vi "AO_single_FPGA.vi"() -> ()   [LabVIEW 2021]
uses:
  <vilib>/rvi/Emulation/niFpgaGetClockAttributes.vi
  <vilib>/rvi/Emulation/niFpgaSctlEmulationGetInTimedLoop.vi
  <vilib>/rvi/Emulation/niFpgaEmulationReportErrorSimple.vi
  <vilib>/rvi/Emulation/niFpgaProcessEmulError.vi
  <vilib>/rvi/interface/RandomDataEmulation/niFpgaRandomDataHandleErrors.vi
  <vilib>/rvi/Emulation/niFpgaCriticalErrorInLSC.vi
  <vilib>/rvi/eio/common/nirviEmuTemplateMethod_errors.vi
  <vilib>/rvi/DataTransferAndStorage/Container/XNode/niFpgaContainer.xnode
  <vilib>/rvi/interface/RandomDataEmulation/nirviRandomDataFpgaReadWriteTemplate.vi
  <vilib>/eio/EIONode/EIONode.xnode
panel:
  in  "AO Enable":bool
  in  "AO 0":sgl
  in  "AO 1":sgl
  in  "AO 2":sgl
  in  "AO 3":sgl
  in  "AO 4":sgl
  in  "AO 5":sgl
  in  "AO 6":sgl
  in  "AO 7":sgl
  in  "AO Loop Timer (ticks)":i32
  out "AO: Actual Loop Rate (ticks)":u32
  out "AO Buffer Underflow?":bool
  in  "AO Buffer Enable":u8 format="%08b"
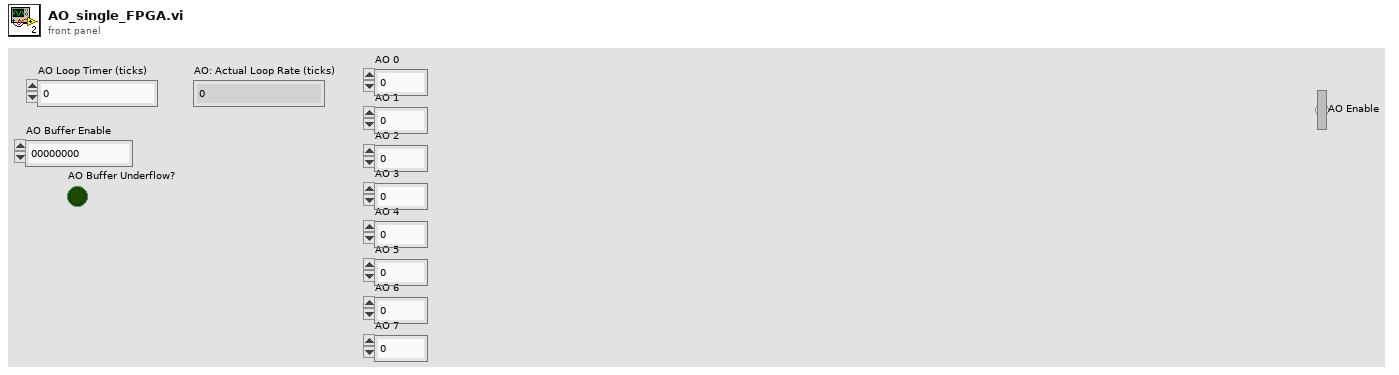
[diagram p1: front panel]
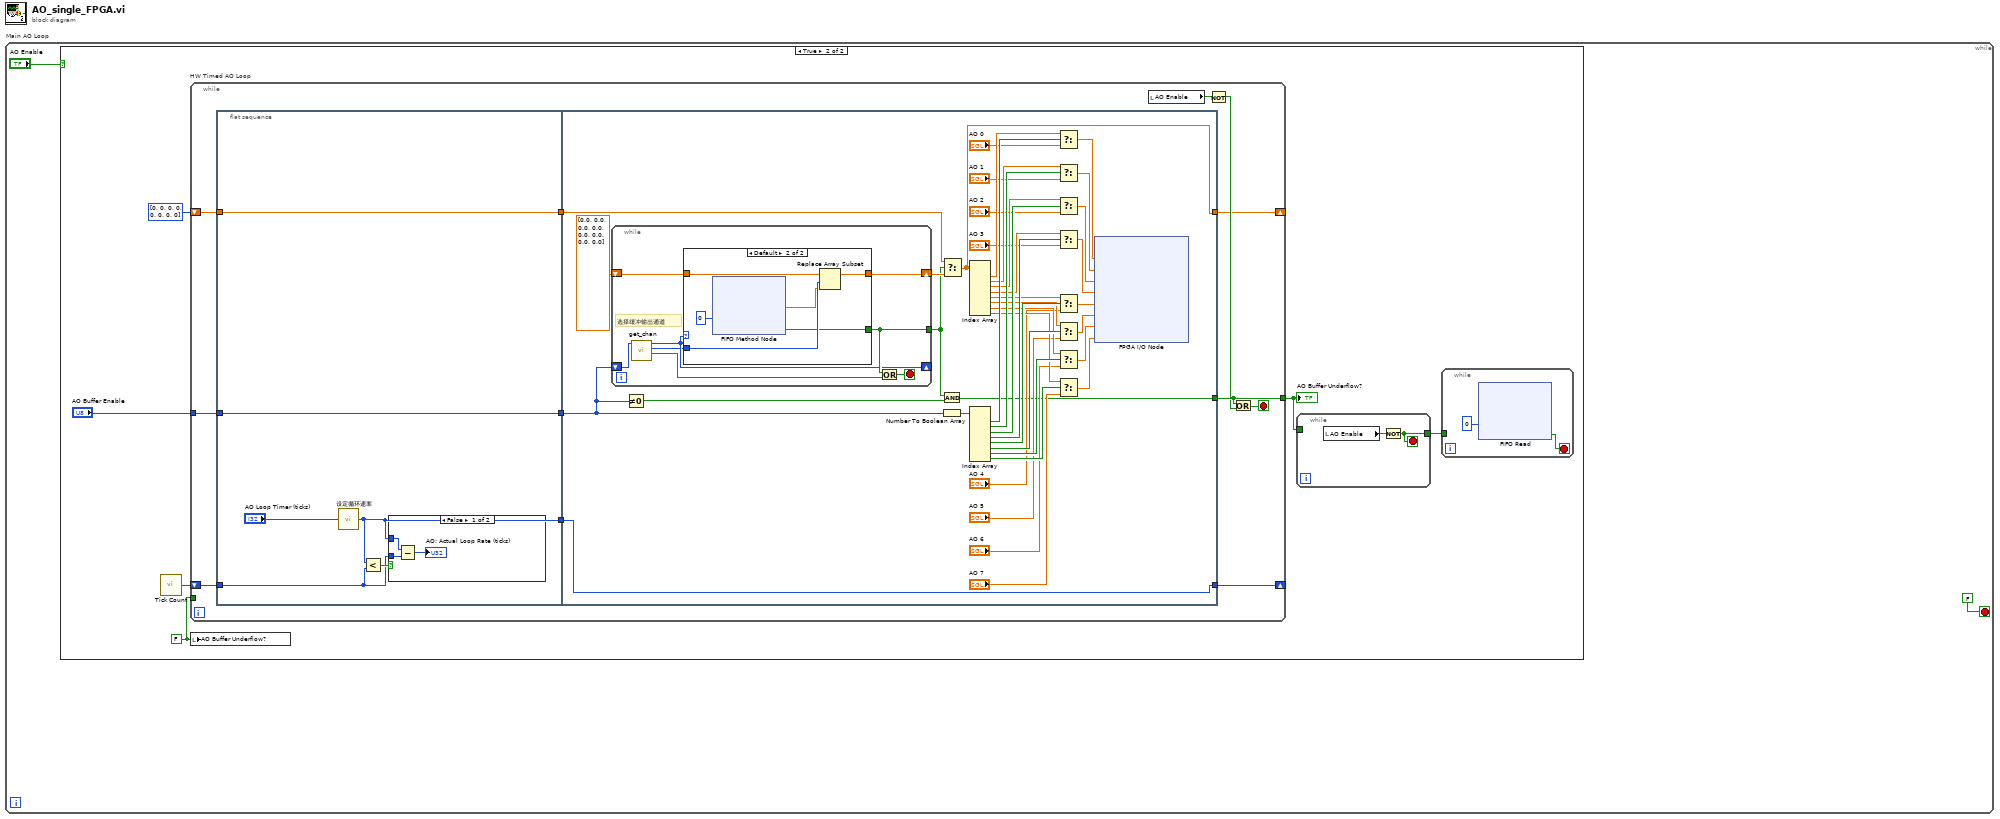
[diagram p0: block diagram]
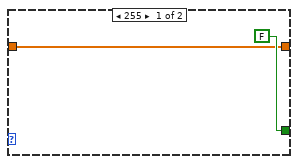
[diagram p4: hidden frame]
diagram:
  n1 = while "Main AO Loop" {
    stop <- FALSE stop-if-true
    n2 = case shown="True" "AO Enable" {
      frame False {
      }
      frame True {
        w8 = FALSE ("AO Buffer Underflow?")
        n3 = call "Tick Count"() -> ("Tick Count(Ticks)"=w3:u32)
        n4 = while "HW Timed AO Loop" {
          tunnel: [w23] -> w5
          tunnel: w8 -> [_]
          tunnel: "AO Buffer Enable" -> [w20]
          shift-right: [w18] -> _
          shift-left: i16[] [0, 0, 0, 0, 0, 0, 0, 0] -> [w17]
          shift-right: [w14] -> _
          shift-left: w3 -> [w13]
          stop <- w24 stop-if-true
          n5 = flat-sequence {
            tunnel: w20 -> [w30]
            tunnel: [w30] -> w19
            tunnel: w17 -> [w29]
            tunnel: [w29] -> w16
            tunnel: [w25] -> w15
            tunnel: w13 -> [w27]
            tunnel: [w34] -> w23
            tunnel: w19 -> [w37]
            tunnel: [w71] -> w18
            tunnel: w16 -> [w70]
            tunnel: w15 -> [w38]
            tunnel: [w38] -> w14
            frame #0 {
              n6 = call "设定循环速率"("Count(Ticks)"="AO Loop Timer (ticks)") -> ("Tick Count(Ticks)"=w25:u32)
              n7 = Less?(x=w25, y=w27) -> (x < y?=w28:bool)
              n8 = case shown="False" w28 {
                tunnel: w25 -> [w33 _]
                tunnel: w27 -> [w32 _]
                frame False {
                  n9 = Subtract(x=w33, y=w32) -> (x-y=→"AO: Actual Loop Rate (ticks)":u32)
                }
                frame True {
                  # "overflow"
                }
              }
            }
            frame #1 {
              n10 = while {
                shift-right: [w82] -> w72
                shift-left: sgl[] [0.0, 0.0, 0.0, 0.0, 0.0, 0.0, 0.0, 0.0] -> [w83]
                tunnel: [w80] -> w35
                shift-right: [w79] -> _
                shift-left: w37 -> [w76]
                stop <- w81 stop-if-true
                # "选择缓冲输出通道"
                n11 = call "get_chan.vi"("AI Select In"=w76) -> ("Stop Loop"=w77:bool, "Current Channel"=w78:u8, "AI Select Out"=w79:u8)  [unwired: 8 in]
                n12 = case shown="Default" w79 {
                  tunnel: w83 -> [w84 w91]
                  tunnel: [w84 w90] -> w82
                  tunnel: [FALSE ("Empty") w87] -> w80
                  tunnel: w78 -> [_ w89]
                  frame 255 {
                  }
                  frame Default {
                    n13 = xnode ("FIFO Method Node")("Timeout"=0) -> ("Element"=w86:sgl, "Timed Out?"=w87:bool)  [unwired: 1 in, 1 out]
                    n14 = Replace Array Subset(array=w91, new element=w86, index=w89) -> (w90:sgl[])
                  }
                }
                n15 = Or(x=w80, y=w77) -> (x .or. y?=w81:bool)
              }
              n16 = Not Equal To 0?(x=w37) -> (x != 0?=w36:bool)
              n17 = And(x=w35, y=w36) -> (x .and. y?=w34:bool)
              n18 = Number To Boolean Array(number=w37) -> (Boolean array=w74:bool[])
              n19 = Select(t=w70, s=w35, f=w72) -> (s? t:f=w71:sgl[])
              n20 = Index Array(array=w71) -> (element #1=w69:sgl, element #2=w66:sgl, element #3=w64:sgl, element #4=w57:sgl, element #5=w50:sgl, element #6=w49:sgl, element #7=w48:sgl, element #8=w47:sgl)  [unwired: 8 in]
              n21 = Index Array(array=w74) -> (element #1=w73:bool, element #2=w67:bool, element #3=w65:bool, element #4=w58:bool, element #5=w54:bool, element #6=w53:bool, element #7=w52:bool, element #8=w51:bool)  [unwired: 8 in]
              n22 = Select(t=w69, s=w73, f="AO 0") -> (s? t:f=w68:sgl)
              n23 = Select(t=w66, s=w67, f="AO 1") -> (s? t:f=w60:sgl)
              n24 = Select(t=w64, s=w65, f="AO 2") -> (s? t:f=w59:sgl)
              n25 = Select(t=w57, s=w58, f="AO 3") -> (s? t:f=w55:sgl)
              n26 = Select(t=w50, s=w54, f="AO 4") -> (s? t:f=w46:sgl)
              n27 = Select(t=w49, s=w53, f="AO 5") -> (s? t:f=w45:sgl)
              n28 = Select(t=w48, s=w52, f="AO 6") -> (s? t:f=w44:sgl)
              n29 = Select(t=w47, s=w51, f="AO 7") -> (s? t:f=w43:sgl)
              n30 = xnode "FPGA I/O Node"("Connector0/AO0"=w68, "Connector0/AO1"=w60, "Connector0/AO2"=w59, "Connector0/AO3"=w55, "Connector0/AO4"=w46, "Connector0/AO5"=w45, "Connector0/AO6"=w44, "Connector0/AO7"=w43) -> ()  [unwired: 8 in, 8 out]
            }
          }
          n31 = local read "AO Enable"() -> (w22:bool)
          n32 = Not(x=w22) -> (.not. x?=w21:bool)
          n33 = Or(x=w23, y=w21) -> (x .or. y?=w24:bool)
        }
        "AO Buffer Underflow?" <- w5
        n34 = local write "AO Buffer Underflow?"(w8) -> ()
        n35 = while {
          tunnel: w5 -> [_]
          tunnel: [w11] -> w4
          stop <- w11 stop-if-true
          n36 = local read "AO Enable"() -> (w12:bool)
          n37 = Not(x=w12) -> (.not. x?=w11:bool)
        }
        n38 = while {
          tunnel: w4 -> [_]
          stop <- w9 stop-if-true
          n39 = xnode ("FIFO Read")("Timeout"=0) -> ("Timed Out?"=w9:bool)  [unwired: 1 in, 2 out]
        }
      }
    }
  }
